vi "TD_Upload_File_Single.vi"(8 "error in (no error)":errorcluster, 9 "file":path, 10 "Upload Url":string, 11 "TekDrive Session In":T1) -> (0 "error out":errorcluster, 3 "TekDrive Session Out":T1)   [LabVIEW 2018]
uses:
  Controls/TekDriveSession.ctl
  <vilib>/httpClient/ClientHandle.ctl
  <vilib>/httpClient/PUTFile.vi
  <vilib>/httpClient/LabVIEWHTTPClient.lvlib
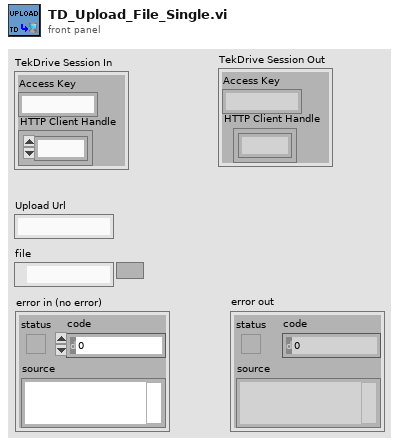
[diagram p1: front panel]
types:
  T1 = typedef "TekDriveSession.ctl" = cluster{"Access Key":string, "HTTP Client Handle":T2}
  T2 = typedef "LabVIEWHTTPClient.lvlib/ClientHandle.ctl" = refnum<k1>
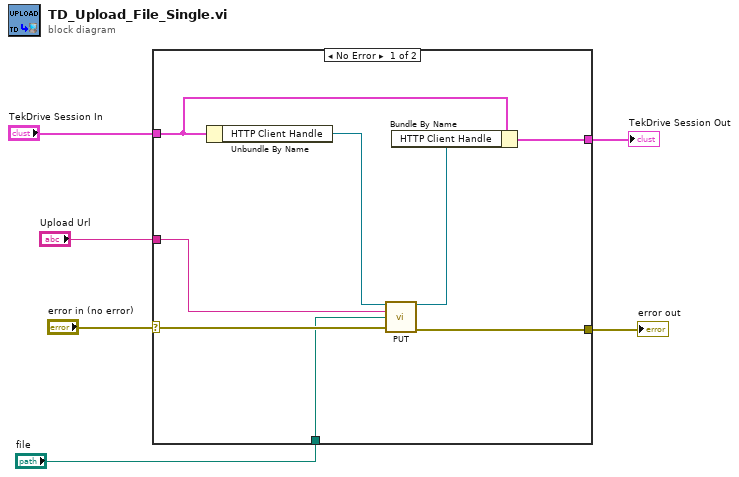
[diagram p0: block diagram]
diagram:
  n1 = case shown="No Error" "error in (no error)" {
    selector: "error in (no error)" -> [w13 w15]
    tunnel: [w14 w15] -> w6
    tunnel: "Upload Url" -> [w12 _]
    tunnel: "TekDrive Session In" -> [w10 w16]
    tunnel: "file" -> [w7 _]
    tunnel: [w8 w16] -> w1
    frame No Error {
      n2 = Unbundle By Name(w10) -> ("HTTP Client Handle"=w11:T2)
      n3 = call-poly <vilib>:"PUT.vi"("client handle"=w11, "url"=w12, "file"=w7, "error in (no error)"=w13) -> ("client handle out"=w9:T2, "error out"=w14:errorcluster)  [unwired: 8 in, 2 out]
      n4 = Bundle By Name(cluster=w10, "HTTP Client Handle"=w9) -> (w8:T1)
    }
    frame Error {
    }
  }
  "error out" <- w6
  "TekDrive Session Out" <- w1
